vi "test Log Span Time.vi"(8 "error in":errorcluster, 11 "TestCase in":refnum<class "Embedded Data Logger System Tests.lvclass">) -> (0 "error out":errorcluster, 3 "TestCase out":refnum<class "Embedded Data Logger System Tests.lvclass">)   [LabVIEW 2018, in "Embedded Data Logger System Tests.lvclass"]
uses:
  Embedded Data Logger System Tests.lvclass
  <vilib>/addons/_JKI Toolkits/VI Tester/TestCase.llb/TestCase.lvclass
  C:/Program Files (x86)/National Instruments/LabVIEW 2018/vi.lib/addons/_JKI Toolkits/VI Tester/TestCase.llb/TestCase.lvclass
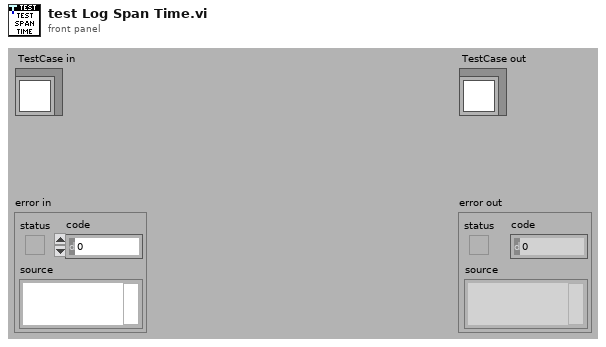
[diagram p1: front panel]
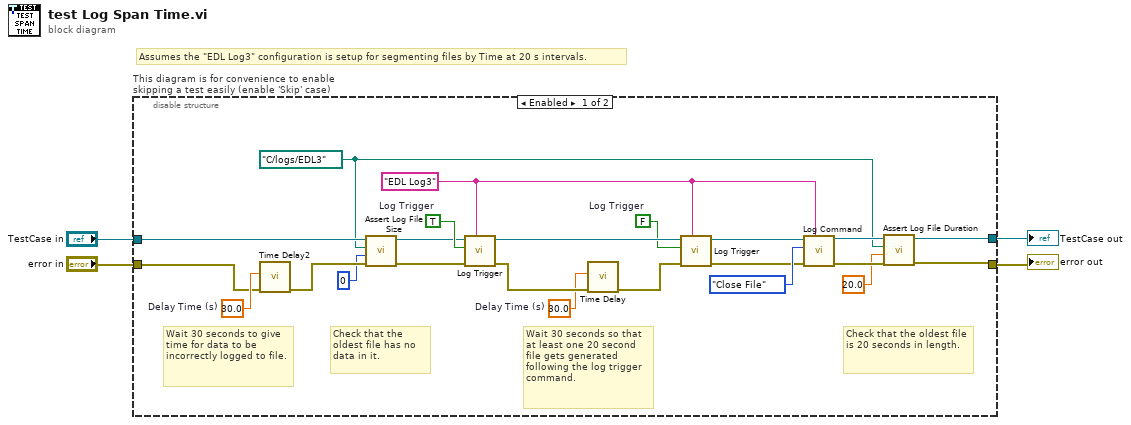
[diagram p0: block diagram]
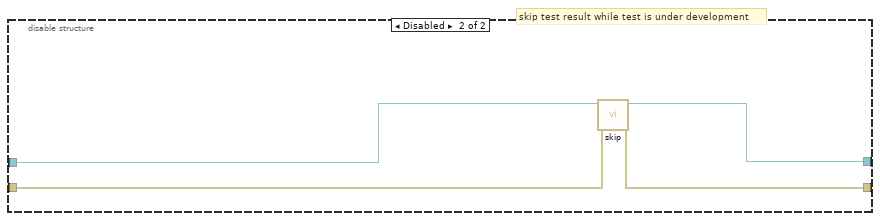
[diagram p2: hidden frame]
diagram:
  # "Assumes the \"EDL Log3\" configuration is setup for segmenting files by Time at 20 s intervals."
  n1 = disable-structure "This diagram is for convenience to enable skipping a test easily (enable 'Skip' case)" shown="Enabled" {
    disable-tunnel: "TestCase in" -> [w9 w30]
    disable-tunnel: [w15 w28] -> w1
    disable-tunnel: [w14 w29] -> w3
    disable-tunnel: "error in" -> [w10 w27]
    frame Enabled {
      w5 = path "C:/logs/EDL3" ("file path")
      w12 = 30.0  # Delay Time (s)
      w13 = "EDL Log3" ("Embedded Data Logger File Name")
      w23 = FALSE  # Log Trigger
      w21 = 30.0  # Delay Time (s)
      w22 = TRUE  # Log Trigger
      # "Check that the oldest file has no data in it."
      # "Wait 30 seconds to give time for data to be incorrectly logged to file."
      # "Check that the oldest file is 20 seconds in length."
      # "Wait 30 seconds so that at least one 20 second file gets generated following the log trigger command."
      n2 = call "Time Delay2"("error in (no error)"=w10, "Delay Time (s)"=w12) -> ("error out"=w11:errorcluster)  [unwired: 9 in]
      n3 = call "Assert Log File Size.vi"("Expected size of file in bytes"=i64 0, "file path"=w5, "Embedded Data Logger System Tests in"=w9) -> ("Embedded Data Logger System Tests out"=w8:refnum<class "Embedded Data Logger System Tests.lvclass">)  [unwired: 7 in, 1 out]
      n4 = call "Log Trigger.vi"("Embedded Data Logger File Name"=w13, "error in"=w11, "Log Trigger"=w22, "Embedded Data Logger System Tests in"=w8) -> ("error out"=w25:errorcluster, "Embedded Data Logger System Tests out"=w24:refnum<class "Embedded Data Logger System Tests.lvclass">)  [unwired: 6 in]
      n5 = call "Time Delay"("error in (no error)"=w25, "Delay Time (s)"=w21) -> ("error out"=w26:errorcluster)  [unwired: 9 in]
      n6 = call "Log Trigger.vi"("Embedded Data Logger File Name"=w13, "error in"=w26, "Log Trigger"=w23, "Embedded Data Logger System Tests in"=w24) -> ("error out"=w19:errorcluster, "Embedded Data Logger System Tests out"=w18:refnum<class "Embedded Data Logger System Tests.lvclass">)  [unwired: 6 in]
      n7 = call "Log Command.vi"("Embedded Data Logger File Name"=w13, "error in"=w19, "Log Command"=enum16{"Idle", "Open File", "Close File"}."Close File", "Embedded Data Logger System Tests in"=w18) -> ("error out"=w17:errorcluster, "Embedded Data Logger System Tests out"=w16:refnum<class "Embedded Data Logger System Tests.lvclass">)  [unwired: 6 in]
      n8 = call "Assert Log File Duration.vi"("error in"=w17, "Expected file duration (s)"=20.0, "File Directory"=w5, "Embedded Data Logger System Tests in"=w16) -> ("error out"=w14:errorcluster, "Embedded Data Logger System Tests out"=w15:refnum<class "Embedded Data Logger System Tests.lvclass">)  [unwired: 6 in]
    }
    frame Disabled {
      # "skip test result while test is under development"
      n9 = call <vilib>:"skip.vi"("error in (no error)"=w27, "TestCase in"=w30) -> ("error out"=w29:errorcluster, "TestCase out"=w28:refnum<class "Embedded Data Logger System Tests.lvclass">)  [unwired: 8 in]
    }
  }
  "error out" <- w3
  "TestCase out" <- w1
